vi "HowHindbraintoMidbrainFilterCalibrate.vi"(3 "HowAmI?":cluster{"T":dbl, "Battery":dbl, "Temp":dbl}) -> (1 "HowAmI? Clean":cluster{"T":dbl, "Battery":dbl, "Temp":dbl})   [LabVIEW 2010]
doc: "This subVI takes raw I16 \"How am I?\" data from the hindbrain and filters and calibrates it to become clean double data for the Midbrain. Cluster is:\n\nt=time\nb=battery"
panel:
  # "This subVI filters and \nand calabrates the\nWhere am I? data \nfrom the hindbrain"
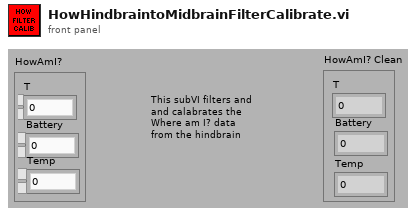
[diagram p1: front panel]
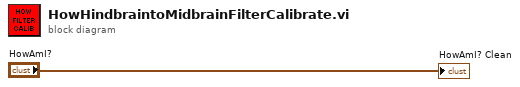
[diagram p0: block diagram]
diagram:
  "HowAmI? Clean" <- "HowAmI?"
